vi "ExamineRawData.vi"() -> ()   [LabVIEW 2024]
uses:
  PreferencesControl.ctl
  <vilib>/Analysis/5stat.llb/RMS (DBL).vi
  <vilib>/Analysis/NI_AALPro.lvlib
panel:
  out "rms value":dbl=10.9322989932631 format="%0.2f"
  out "Plots":T1={"Hammer"=[{0.0, "dt"=2.0833333333333333e-05, "Y"=array[14400 elements]}], "Microphone"=[{0.0, "dt"=2.0833333333333333e-05, "Y"=array[14400 elements]}], "Hammer Spectrum"=[{0.0, "dt"=1.0, "Y"=array[24000 elements]}, {0.0, "dt"=1.0, "Y"=array[24000 elements]}, {0.0, "dt"=1.0, "Y"=array[24000 elements]}, {0.0, "dt"=1.0, "Y"=array[24000 elements]}, {0.0, "dt"=1.0, "Y"=array[24000 elements]}], "FRF"=[{0.0, "dt"=1.0, "Y"=array[24000 elements]}, {0.0, "dt"=1.0, "Y"=array[24000 elements]}]}
  in  "View":u16(ring)=2 items=["Raw", "Volts", "Units (Pa, N, etc)"]
  in  "Settings":T2={"Name of test"="Vibrometer--Vibrometer 1", "Date"=timestamp(3619802663 s since 1904-01-01), "Location"="Home", "Template"="ScratchPad", "Soundcard"="OCTA-CAPTURE", "resolution"=32, "Sampling rate"=48000, "Ch1 Gain "=20.0, "Ch2 Gain"=20.0, "Sample time (s)"=0.3, "Pre-trigger (s)"=0.001, "Hammer Threshold"=0.01, "Positions"=1, "Taps/Position"=5, "Set Names"="H", "Freq resolution"=1.0, "Hammer cutoff"=0.025, "Mic cutoff"=0.25, "Double bounce "=0.01, "Hammer Cal"=1.0, "dB Offset"=0.0, "Accel Cal"=1.0, "Vibrometer Cal"=40.0, "Mic Cal"=49.38, "Output"=3, "Voltage Cal"=13.8, "Vibrometer Port"="ASRL27::INSTR", "Range"=50, "High Pass"=2, "Bandwidth"=25, "X Range"=[], "Y Range"=[], "dB Spread"=0.0, "Trigger"=0, "Ch_1"=1, "Ch_2"=2, "flip?"=FALSE, "60Hz"=FALSE, "Time offset"=0.0, "Piezo Cal"=1.0, "Default Notes"=""} {"Ch_2" min=1 step=1; "Ch_1" min=1 max=100 step=1; "Trigger" items=["Hammer (force)", "Self-tap", "Spacebar"]; "Bandwidth" items=["1 kHz"=1, "5 kHz"=5, "10 kHz"=10, "25 kHz"=25, "50 kHz"=50, "100 kHz"=100]; "High Pass" items=["Off", "13 Hz", "104 Hz"]; "Range" items=["10 mm/s"=1, "20 mm/s"=2, "50 mm/s"=5, "100 mm/s"=10, "200 mm/s"=20, "500 mm/s"=50, "1 m/s"=100, "2 m/s"=200]; "Output" items=["Accelerometer", "Speed (from acceleration)", "Microphone", "Vibrometer", "Piezo"]; "Voltage Cal" format="%#_13g"; "Ch2 Gain" format="%#_13g"; "Ch1 Gain" format="%#_13g"; "Double bounce" min=0.0; "Mic cutoff" min=0.0 format="%#_4g"; "Hammer cutoff" min=0.0 format="%#_4g"; "Freq resolution" min=0.0; "Pre-trigger (s)" format="%#_13g"; "Date" format="%<%H:%M\n%d/%m/%y>T"; "resolution" items=["16 bit"=16, "24 bit"=24, "32 bit"=32]; "Sampling rate" items=["22050 samp/s"=22050, "44100 samp/s"=44100, "48000 samp/s"=48000]}
  # "Hz"
  # "dB"
  # "dB"
  # "sec"
  # "sec"
  # "mV/Pa"
  # "mV/m/s2"
  # "mV/mm/s"
  # "V/N"
  # "sec"
  # "sec"
  # "mV/N"
  # "a.u."
  # "a.u."
  # "sec"
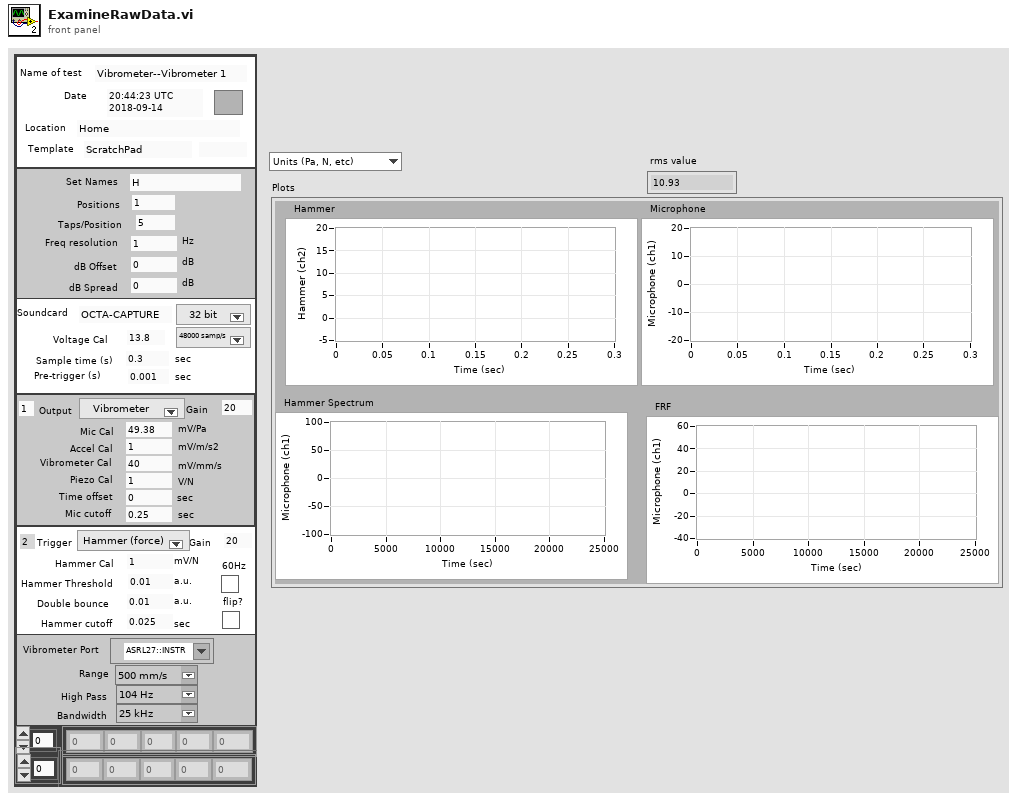
[diagram p1: front panel]
types:
  T1 = cluster{"Hammer":cluster{dbl, "dt":dbl, "Y":dbl[]}[], "Microphone":cluster{dbl, "dt":dbl, "Y":dbl[]}[], "Hammer Spectrum":cluster{dbl, "dt":dbl, "Y":dbl[]}[], "FRF":cluster{dbl, "dt":dbl, "Y":dbl[]}[]}
  T2 = typedef "PreferencesControl.ctl" = cluster{"Name of test":string, "Date":timestamp, "Location":string, "Template":string, "Soundcard":string, "resolution":u16, "Sampling rate":u16, "Ch1 Gain ":dbl, "Ch2 Gain":dbl, "Sample time (s)":dbl, "Pre-trigger (s)":dbl, "Hammer Threshold":dbl, "Positions":i16, "Taps/Position":i16, "Set Names":string, "Freq resolution":dbl, "Hammer cutoff":dbl, "Mic cutoff":dbl, "Double bounce ":dbl, "Hammer Cal":dbl, "dB Offset":dbl, "Accel Cal":dbl, "Vibrometer Cal":dbl, "Mic Cal":dbl, "Output":u16, "Voltage Cal":dbl, "Vibrometer Port":refnum<visa-resource-name>, "Range":u16, "High Pass":u16, "Bandwidth":u16, "X Range":cluster{"Minimum":dbl, "Maximum":dbl, "Increment":dbl, "Minor Increment":dbl, "Start":dbl}[], "Y Range":cluster{"Minimum":dbl, "Maximum":dbl, "Increment":dbl, "Minor Increment":dbl, "Start":dbl}[], "dB Spread":dbl, "Trigger":u16, "Ch_1":u8, "Ch_2":u8, "flip?":bool, "60Hz":bool, "Time offset":dbl, "Piezo Cal":dbl, "Default Notes":string}
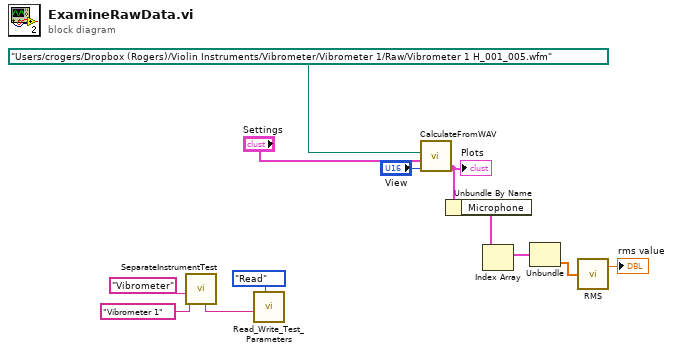
[diagram p0: block diagram]
diagram:
  n1 = call "SeparateInstrumentTest.vi"("test in"="Vibrometer 1" ("Instrument"), "Instrument in"="Vibrometer" ("Instrument")) -> ("Instrument -- test out"=w11:string)  [unwired: 5 in, 4 out]
  n2 = call "Read_Write_Test_Parameters.vi"("Task"=enum16{"Save", "Read", "Clear"}."Read", "Instrument Name"=w11) -> ()  [unwired: 8 in, 2 out]
  n3 = call "CalculateFromWAV.vi"("View"="View", "Settings"="Settings", "path"=path "/Users/crogers/Dropbox (Rogers)/Violin Instruments/Vibrometer/Vibrometer 1/Raw/Vibrometer 1 H_001_005.wfm" ("appended path")) -> ("Plots"=w5:T1)  [unwired: 4 in, 4 out]
  "Plots" <- w5
  n4 = Unbundle By Name(w5) -> ("Microphone"=w4:cluster{dbl, "dt":dbl, "Y":dbl[]}[])
  n5 = Index Array(array=w4) -> (element=w3:cluster{dbl, "dt":dbl, "Y":dbl[]})  [unwired: 1 in]
  n6 = Unbundle(w3) -> ("Y"=w2:dbl[])  [unwired: 2 out]
  n7 = call-poly <vilib>:"RMS.vi"("X"=w2) -> ("rms value"=→"rms value":dbl)  [unwired: 1 out]
